vi "Send and recieve string.vi"() -> ()   [LabVIEW 2011]
uses:
  <vilib>/LabVIEW Interface for Arduino/Type Defs/Connection Type.ctl
  <vilib>/LabVIEW Interface for Arduino/Type Defs/Board Type.ctl
  <vilib>/LabVIEW Interface for Arduino/LabVIEW Interface for Arduino.lvlib
panel:
  in  "Tab Control":enum32{"Settings", "Page 2"}(tab)
  in  "VISA resource name":refnum<visa-resource-name>
  in  "Baud Rate":u32
  in  "Connection Type":T1
  in  "Board Type":T2
  out "Error Out":errorcluster
  out "String 2":string
  in  "String":string
  in  "Stop Button":bool
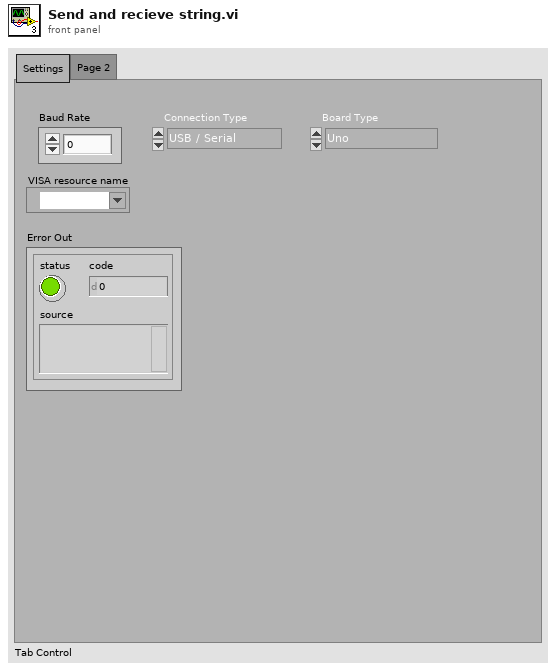
[diagram p1: front panel]
types:
  T1 = typedef "LabVIEW Interface for Arduino.lvlib/Connection Type.ctl" = enum8{"USB / Serial", "XBEE", "BlueSmirf (Bluetooth)"}
  T2 = typedef "LabVIEW Interface for Arduino.lvlib/Board Type.ctl" = enum16{"Uno", "Dimuelanove w/Atmega 328", "Mega 2560"}
  T3 = typedef "LabVIEW Interface for Arduino.lvlib/Arduino Resource.ctl" = cluster{"VISA resource":refnum<visa-resource-name>, "Board Type":T2, "Connection Type":enum8{"USB / Serial"}, "Bytes Per Packet (15)":u8}
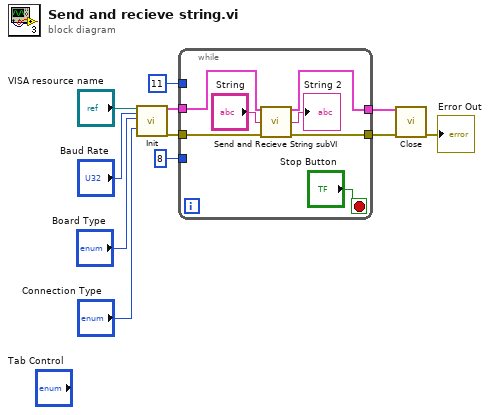
[diagram p0: block diagram]
diagram:
  n1 = call <vilib>:"Init.vi"("VISA resource"="VISA resource name", "Baud Rate (115200)"="Baud Rate", "Board Type (Uno)"="Board Type", "Connection Type (USB/Serial)"="Connection Type") -> ("Arduino Resource"=w8:T3, "error out"=w7:errorcluster)  [unwired: 14 in]
  n2 = while {
    tunnel: w8 -> [w17]
    tunnel: w7 -> [w16]
    tunnel: 11 -> [_]
    tunnel: 8 -> [_]
    tunnel: [w13] -> w2
    tunnel: [w12] -> w1
    stop <- "Stop Button" stop-if-true
    n3 = call "Send and Recieve String subVI.vi"("Arduino Resource"=w17, "String"="String", "error in"=w16) -> ("Arduino Resource 2"=w13:T3, "String Output"=→"String 2":string, "error out"=w12:errorcluster)  [unwired: 10 in]
  }
  n4 = call <vilib>:"Close.vi"("Arduino Resource"=w2, "error in"=w1) -> ("error out"=→"Error Out":errorcluster)  [unwired: 13 in]
